vi "Update Polygon Marker Position.vi"(8 "Error In":errorcluster, 10 "index":i32, 11 "This VI":refnum<vi>) -> (0 "error out":errorcluster)   [LabVIEW 2014]
uses:
  C:/Robotic Systems/Products/AgFalcon/Software/Ground Station/Data/Mapping DLL/GMap.NET.WindowsForms.dll
  Data/Mapping DLL/GMap.NET.WindowsForms.dll
  Reference/SubVI/Main Map Control Refernce.vi
  Reference/SubVI/GMap DLL Refernce.vi
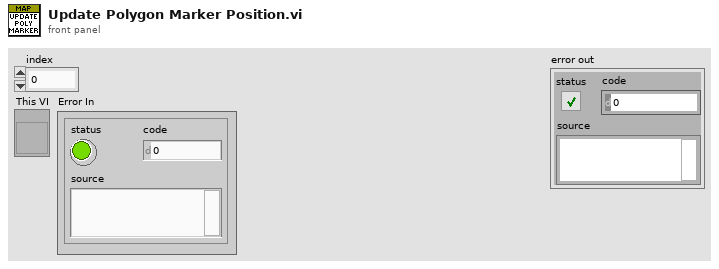
[diagram p1: front panel]
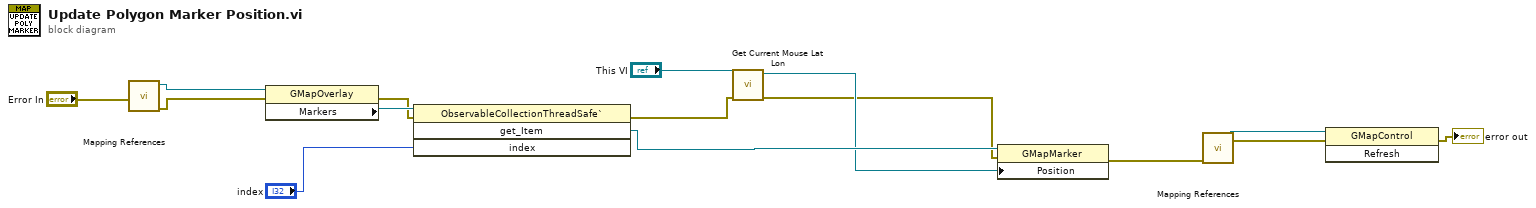
[diagram p0: block diagram]
diagram:
  n1 = call-poly "Mapping References.vi"("Error In"="Error In") -> ("Error Out"=w14:errorcluster, "Main Map Reference"=w15:refnum<k24>)  [unwired: 9 in]
  n2 = property class="GMapOverlay"(reference=w15, error in=w14) -> (error out=w12:errorcluster, "Markers"=w13:refnum<k24>)  [unwired: 1 out]
  n3 = invoke class="ObservableCollectionThreadSafe`" method="get_Item"(reference=w13, error in=w12, "index"="index") -> (error out=w3:errorcluster, "get_Item"=w9:refnum<k24>)  [unwired: 1 in, 2 out]
  n4 = call "Get Current Mouse Lat Lon.vi"("error in (no error)"=w3, "This VI"="This VI") -> ("Error Out"=w2:errorcluster, "Point Ref"=w8:refnum<k24>)  [unwired: 6 in, 2 out]
  n5 = property class="GMapMarker"(reference=w9, error in=w2, "Position"=w8) -> (error out=w1:errorcluster)  [unwired: 1 out]
  n6 = call-poly "Mapping References.vi"("Error In"=w1) -> ("Error Out"=w6:errorcluster, "GMap DLL Reference"=w5:refnum<k24>)  [unwired: 9 in]
  n7 = invoke class="GMapControl" method="Refresh"(reference=w5, error in=w6) -> (error out=→"error out":errorcluster)  [unwired: 1 in, 2 out]
